vi "evlmem03.vi"(1 "fdt":dbl, 2 "xms":dbl, 3 "d":dbl[](array[numeric])) -> (0 "P":dbl)   [LabVIEW 2015]
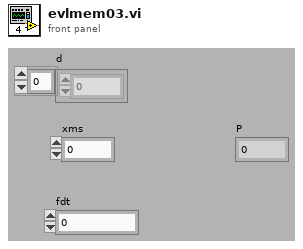
[diagram p1: front panel]
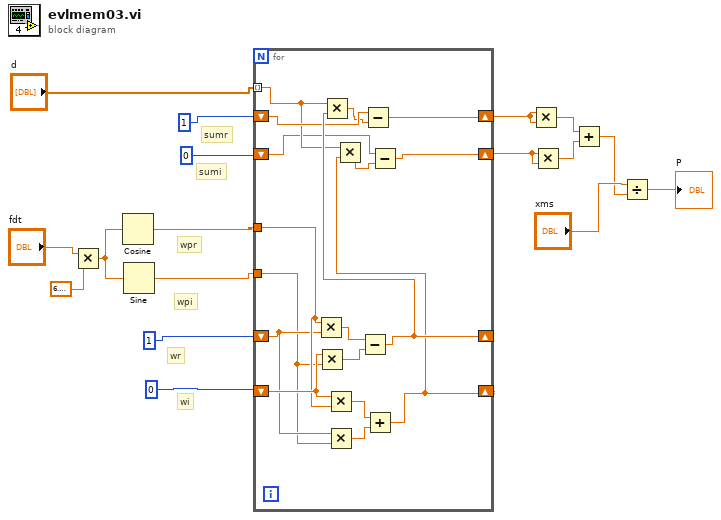
[diagram p0: block diagram]
diagram:
  # "sumi"
  # "sumr"
  # "wi"
  # "wr"
  # "wpi"
  # "wpr"
  n1 = Multiply(x="fdt", y=6.283185307179586) -> (x*y=w15:dbl)
  n2 = Cosine(x=w15) -> (cos(x)=w12:dbl)
  n3 = Sine(x=w15) -> (sin(x)=w11:dbl)
  n4 = for {
    tunnel: "d" -> [w22] mode=indexing
    shift-right: [w26] -> _
    shift-left: 1 -> [w30]
    tunnel: w12 -> [w31]
    tunnel: w11 -> [w29]
    shift-right: [w21] -> _
    shift-left: 0 -> [w32]
    shift-right: [w23] -> w7
    shift-left: 1 -> [w25]
    shift-right: [w18] -> w6
    shift-left: 0 -> [w20]
    n5 = Multiply(x=w31, y=w30) -> (x*y=w34:dbl)
    n6 = Multiply(x=w32, y=w29) -> (x*y=w33:dbl)
    n7 = Multiply(x=w32, y=w31) -> (x*y=w28:dbl)
    n8 = Multiply(x=w30, y=w29) -> (x*y=w27:dbl)
    n9 = Subtract(x=w34, y=w33) -> (x-y=w26:dbl)
    n10 = Multiply(x=w22, y=w26) -> (x*y=w24:dbl)
    n11 = Subtract(x=w25, y=w24) -> (x-y=w23:dbl)
    n12 = Add(x=w28, y=w27) -> (x+y=w21:dbl)
    n13 = Multiply(x=w22, y=w21) -> (x*y=w19:dbl)
    n14 = Subtract(x=w20, y=w19) -> (x-y=w18:dbl)
  }
  n15 = Multiply(x=w7, y=w7) -> (x*y=w5:dbl)
  n16 = Multiply(x=w6, y=w6) -> (x*y=w4:dbl)
  n17 = Add(x=w5, y=w4) -> (x+y=w2:dbl)
  n18 = Divide(x="xms", y=w2) -> (x/y=→"P":dbl)
